vi "Bool_Delay Out.vi"(5 "Off Delay (S)":dbl format="%.3g", 7 "On Delay (S)":dbl format="%.3g", 10 "Initial State In":bool, 11 "input In":bool) -> (3 "Delayed Output Out":bool)   [LabVIEW 2020]
panel:
  in  "stop":bool=TRUE
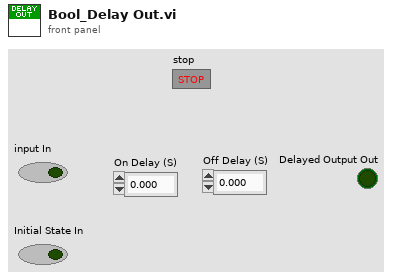
[diagram p1: front panel]
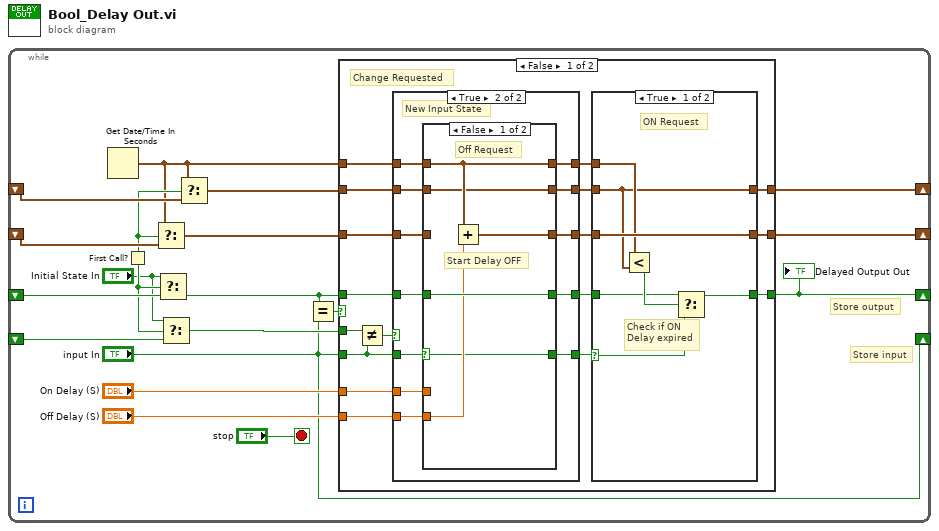
[diagram p0: block diagram]
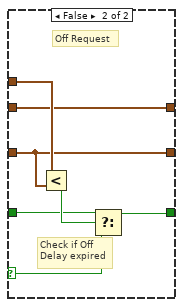
[diagram p2: hidden frame]
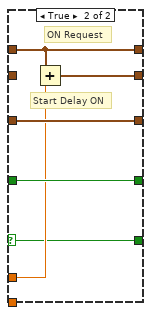
[diagram p4: hidden frame]
diagram:
  n1 = while {
    shift-right: [w13] -> _
    shift-left: _ -> [w18]
    shift-right: [w15] -> _
    shift-left: _ -> [w17]
    shift-right: [w6] -> _
    shift-left: _ -> [w12]
    shift-right: ["input In"] -> _
    shift-left: _ -> [w8]
    stop <- "stop" stop-if-true
    # "Store output"
    # "Store input"
    n2 = Get Date/Time In Seconds() -> (seconds since 1Jan1904=w5:timestamp)
    n3 = First Call?() -> (First Call?: T/F=w9:bool)
    n4 = Select(t=w5, s=w9, f=w17) -> (s? t:f=w16:timestamp)
    n5 = Select(t="Initial State In", s=w9, f=w12) -> (s? t:f=w11:bool)
    n6 = Select(t="Initial State In", s=w9, f=w8) -> (s? t:f=w7:bool)
    n7 = Select(t=w5, s=w9, f=w18) -> (s? t:f=w14:timestamp)
    n8 = Equal?(x=w11, y="input In") -> (x = y?=w10:bool)
    n9 = case shown="False" w10 {
      tunnel: [w22 w82] -> w15
      tunnel: w16 -> [w34 w82]
      tunnel: w14 -> [w35 w81]
      tunnel: [w23 w81] -> w13
      tunnel: [w20 w80] -> w6
      tunnel: w11 -> [w33 w80]
      tunnel: "On Delay (S)" -> [w29 _]
      tunnel: "Off Delay (S)" -> [w28 _]
      tunnel: "input In" -> [w30 _]
      tunnel: w7 -> [w36 _]
      tunnel: w5 -> [w32 _]
      frame False {
        # "Change Requested"
        n10 = Not Equal?(x=w36, y=w30) -> (x != y?=w31:bool)
        n11 = case shown="True" w31 {
          tunnel: w35 -> [w52 w66]
          tunnel: [w52 w60] -> w25
          tunnel: w34 -> [w53 w65]
          tunnel: [w53 w59] -> w26
          tunnel: w33 -> [w54 w64]
          tunnel: [w54 w58] -> w21
          tunnel: w32 -> [w51 w67]
          tunnel: w30 -> [w55 w63]
          tunnel: w29 -> [_ w62]
          tunnel: w28 -> [_ w61]
          tunnel: [w55 w57] -> w27
          tunnel: [w51 w56] -> w24
          frame False {
            # "Same Input state"
          }
          frame True {
            # "New Input State"
            n12 = case shown="False" w63 {
              selector: w63 -> [w68 w75]
              tunnel: w67 -> [w73 w74]
              tunnel: w66 -> [w72 _]
              tunnel: w65 -> [_ w79]
              tunnel: w64 -> [w71 w78]
              tunnel: w62 -> [_ w76]
              tunnel: w61 -> [w69 _]
              tunnel: [w72 w77] -> w60
              tunnel: [w70 w79] -> w59
              tunnel: [w71 w78] -> w58
              tunnel: [w68 w75] -> w57
              tunnel: [w73 w74] -> w56
              frame False {
                # "Off Request"
                # "Start Delay OFF"
                n13 = Add(x=w73, y=w69) -> (x+y=w70:timestamp)
              }
              frame True {
                # "ON Request"
                # "Start Delay ON"
                n14 = Add(x=w74, y=w76) -> (x+y=w77:timestamp)
              }
            }
          }
        }
        n15 = case shown="True" w27 {
          selector: w27 -> [w37 w45]
          tunnel: w26 -> [w43 w44]
          tunnel: w25 -> [w41 w49]
          tunnel: w24 -> [w42 w50]
          tunnel: [w41 w49] -> w23
          tunnel: [w43 w44] -> w22
          tunnel: w21 -> [w39 w47]
          tunnel: [w38 w46] -> w20
          frame True {
            # "ON Request"
            # "Check if ON\nDelay expired"
            n16 = Less?(x=w42, y=w41) -> (x < y?=w40:bool)
            n17 = Select(t=w39, s=w40, f=w37) -> (s? t:f=w38:bool)
          }
          frame False {
            # "Off Request"
            # "Check if Off\nDelay expired"
            n18 = Less?(x=w50, y=w44) -> (x < y?=w48:bool)
            n19 = Select(t=w47, s=w48, f=w45) -> (s? t:f=w46:bool)
          }
        }
      }
      frame True {
        # "No change requested"
      }
    }
    "Delayed Output Out" <- w6
  }
